vi "VI Tree.vi"   [LabVIEW 2015, in "Agilent 2000 3000 X-Series.lvlib"]
doc: "This is the instrument driver for the Agilent 2000 3000 X-Series oscilloscope. The VI Tree displays all the user-callable VIs of the instrument driver in an organized table."
uses:
  <instrlib>/Agilent 2000 3000 X-Series/Agilent 2000 3000 X-Series.lvlib
  <instrlib>/Agilent 2000 3000 X-Series/Public/Configure/Configure Timebase (Basic).vi
  <instrlib>/Agilent 2000 3000 X-Series/Public/Configure/Configure Measurement Edge (Delay).vi
  <instrlib>/Agilent 2000 3000 X-Series/Public/Action-Status/Reset Count (Mask Test).vi
  <instrlib>/Agilent 2000 3000 X-Series/Public/Configure/Trigger/Configure Trigger (USB).vi
  <instrlib>/Agilent 2000 3000 X-Series/Public/Configure/Serial Bus/Configure Serial Bus (IIC - Trigger).vi
  <instrlib>/Agilent 2000 3000 X-Series/Public/Configure/Reference Waveform/Configure Reference Waveform (Operation).vi
  <instrlib>/Agilent 2000 3000 X-Series/Public/Configure/Math/Configure Math Function (Bus).vi
  <instrlib>/Agilent 2000 3000 X-Series/Public/Configure/Mask Test/Configure Mask Test (Measurement).vi
  <instrlib>/Agilent 2000 3000 X-Series/Public/Configure/Digital Bus/Configure Bus Definition (Bits Mask).vi
  <instrlib>/Agilent 2000 3000 X-Series/Public/Data/Read Waveforms (Single).vi
  <instrlib>/Agilent 2000 3000 X-Series/Public/Data/Read Measurement (Current Value).vi
  <instrlib>/Agilent 2000 3000 X-Series/Public/Data/Read Count Measurement (Event Search).vi
  <instrlib>/Agilent 2000 3000 X-Series/Public/Configure/Event Search/Configure Event Search (Serial Bus - SENT).vi
  <instrlib>/Agilent 2000 3000 X-Series/Public/Configure/Waveform Modulation/Configure Waveform Modulation (AM).vi
  <instrlib>/Agilent 2000 3000 X-Series/Public/Configure/Power Analysis/Configure Power Analysis (Efficiency).vi
  <instrlib>/Agilent 2000 3000 X-Series/Public/Configure/Math/Configure Clock Recovery (Constant Frequency).vi
  <instrlib>/Agilent 2000 3000 X-Series/Public/Data/Read Jitter Measurement (Clock TIE).vi
  <instrlib>/Agilent 2000 3000 X-Series/Public/Configure/Jitter Analysis/Configure Jitter Measurement (N-Period to Period).vi
panel:
  # "(c) 2011-2016 National Instruments.  ALL RIGHTS RESERVED."
  # "SEE DIAGRAM\nFOR VI TREE."
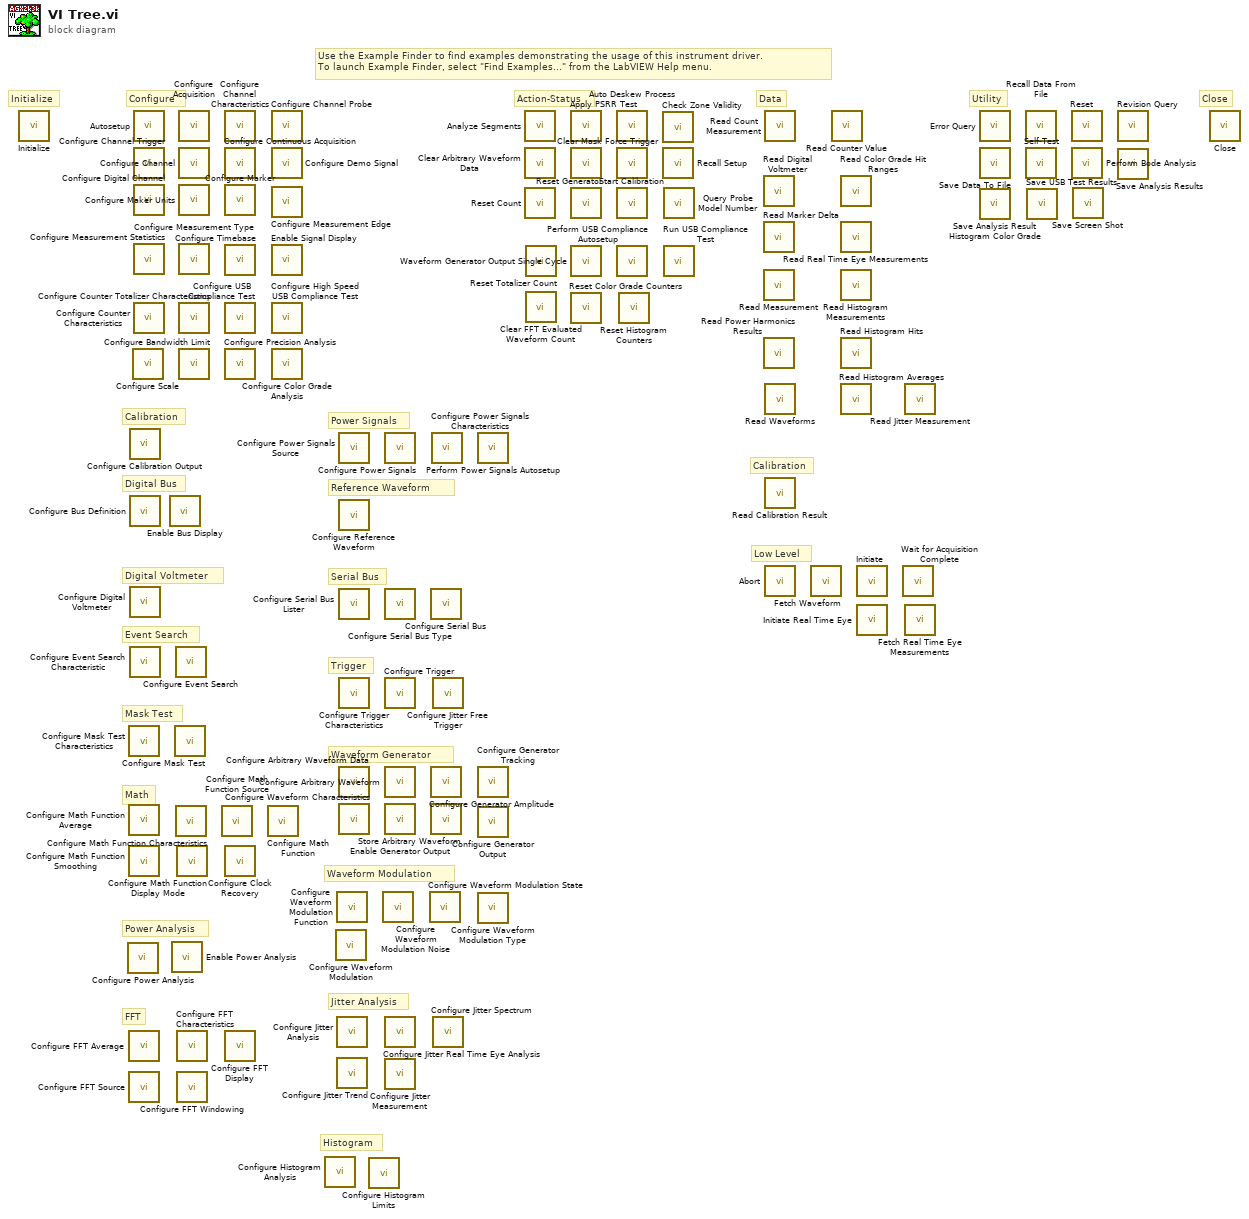
[diagram p0: block diagram]
diagram:
  # "Histogram"
  # "Jitter Analysis"
  # "FFT"
  # "Waveform Modulation"
  # "Digital Voltmeter"
  # "Close"
  # "Utility"
  # "Power Analysis"
  # "Low Level"
  # "Calibration"
  # "Data"
  # "Waveform Generator"
  # "Trigger"
  # "Serial Bus"
  # "Reference Waveform"
  # "Power Signals"
  # "Math"
  # "Mask Test"
  # "Event Search"
  # "Digital Bus"
  # "Calibration"
  # "Configure"
  # "Action-Status"
  # "Initialize"
  # "Use the Example Finder to find examples demonstrating the usage of this instrument driver.\nTo launch Example Finder, select \"Find Examples...\" from the LabVIEW Help menu."
  n1 = call <instrlib>:"Initialize.vi"() -> ()  [unwired: 10 in, 2 out]
  n2 = call-poly <instrlib>:"Configure Power Analysis.vi"() -> ()  [unwired: 10 in, 2 out]
  n3 = call <instrlib>:"Configure Mask Test Characteristics.vi"() -> ()  [unwired: 14 in, 2 out]
  n4 = call <instrlib>:"Configure Math Function Average.vi"() -> ()  [unwired: 10 in, 2 out]
  n5 = call <instrlib>:"Configure Math Function Smoothing.vi"() -> ()  [unwired: 10 in, 2 out]
  n6 = call <instrlib>:"Configure FFT Average.vi"() -> ()  [unwired: 10 in, 2 out]
  n7 = call <instrlib>:"Configure FFT Source.vi"() -> ()  [unwired: 10 in, 2 out]
  n8 = call <instrlib>:"Configure Calibration Output.vi"() -> ()  [unwired: 10 in, 2 out]
  n9 = call-poly <instrlib>:"Configure Bus Definition.vi"() -> ()  [unwired: 10 in, 2 out]
  n10 = call <instrlib>:"Configure Digital Voltmeter.vi"() -> ()  [unwired: 10 in, 2 out]
  n11 = call <instrlib>:"Configure Event Search Characteristic.vi"() -> ()  [unwired: 10 in, 2 out]
  n12 = call <instrlib>:"Configure Scale.vi"() -> ()  [unwired: 10 in, 2 out]
  n13 = call <instrlib>:"Autosetup.vi"() -> ()  [unwired: 10 in, 2 out]
  n14 = call <instrlib>:"Configure Channel Trigger.vi"() -> ()  [unwired: 10 in, 2 out]
  n15 = call <instrlib>:"Configure Digital Channel.vi"() -> ()  [unwired: 10 in, 2 out]
  n16 = call <instrlib>:"Configure Measurement Statistics.vi"() -> ()  [unwired: 10 in, 2 out]
  n17 = call <instrlib>:"Configure Counter Characteristics.vi"() -> ()  [unwired: 14 in, 2 out]
  n18 = call <instrlib>:"Enable Bus Display.vi"() -> ()  [unwired: 10 in, 2 out]
  n19 = call <instrlib>:"Enable Power Analysis.vi"() -> ()  [unwired: 10 in, 2 out]
  n20 = call-poly <instrlib>:"Configure Mask Test.vi"() -> ()  [unwired: 14 in, 2 out]
  n21 = call-poly <instrlib>:"Configure Event Search.vi"() -> ()  [unwired: 10 in, 2 out]
  n22 = call <instrlib>:"Configure Math Function Characteristics.vi"() -> ()  [unwired: 14 in, 2 out]
  n23 = call <instrlib>:"Configure Math Function Display Mode.vi"() -> ()  [unwired: 10 in, 2 out]
  n24 = call <instrlib>:"Configure FFT Characteristics.vi"() -> ()  [unwired: 14 in, 2 out]
  n25 = call <instrlib>:"Configure FFT Windowing.vi"() -> ()  [unwired: 10 in, 2 out]
  n26 = call <instrlib>:"Configure Acquisition.vi"() -> ()  [unwired: 10 in, 2 out]
  n27 = call <instrlib>:"Configure Channel.vi"() -> ()  [unwired: 14 in, 2 out]
  n28 = call <instrlib>:"Configure Maker Units.vi"() -> ()  [unwired: 10 in, 2 out]
  n29 = call <instrlib>:"Configure Measurement Type.vi"() -> ()  [unwired: 14 in, 2 out]
  n30 = call <instrlib>:"Configure Counter Totalizer Characteristics.vi"() -> ()  [unwired: 14 in, 2 out]
  n31 = call <instrlib>:"Configure Bandwidth Limit.vi"() -> ()  [unwired: 10 in, 2 out]
  n32 = call <instrlib>:"Configure Math Function Source.vi"() -> ()  [unwired: 10 in, 2 out]
  n33 = call <instrlib>:"Configure Channel Characteristics.vi"() -> ()  [unwired: 10 in, 2 out]
  n34 = call <instrlib>:"Configure Continuous Acquisition.vi"() -> ()  [unwired: 10 in, 2 out]
  n35 = call <instrlib>:"Configure Marker.vi"() -> ()  [unwired: 14 in, 2 out]
  n36 = call-poly <instrlib>:"Configure Timebase.vi"() -> ()  [unwired: 14 in, 2 out]
  n37 = call <instrlib>:"Configure USB Compliance Test.vi"() -> ()  [unwired: 10 in, 2 out]
  n38 = call <instrlib>:"Configure Precision Analysis.vi"() -> ()  [unwired: 10 in, 2 out]
  n39 = call-poly <instrlib>:"Configure Clock Recovery.vi"() -> ()  [unwired: 10 in, 2 out]
  n40 = call <instrlib>:"Configure FFT Display.vi"() -> ()  [unwired: 10 in, 2 out]
  n41 = call-poly <instrlib>:"Configure Math Function.vi"() -> ()  [unwired: 10 in, 2 out]
  n42 = call <instrlib>:"Configure Channel Probe.vi"() -> ()  [unwired: 10 in, 2 out]
  n43 = call <instrlib>:"Configure Demo Signal.vi"() -> ()  [unwired: 10 in, 2 out]
  n44 = call-poly <instrlib>:"Configure Measurement Edge.vi"() -> ()  [unwired: 10 in, 2 out]
  n45 = call <instrlib>:"Enable Signal Display.vi"() -> ()  [unwired: 10 in, 2 out]
  n46 = call <instrlib>:"Configure High Speed USB Compliance Test.vi"() -> ()  [unwired: 10 in, 2 out]
  n47 = call <instrlib>:"Configure Color Grade Analysis .vi"() -> ()  [unwired: 10 in, 2 out]
  n48 = call <instrlib>:"Configure Histogram Analysis.vi"() -> ()  [unwired: 10 in, 2 out]
  n49 = call-poly <instrlib>:"Configure Waveform Modulation.vi"() -> ()  [unwired: 10 in, 2 out]
  n50 = call <instrlib>:"Configure Waveform Modulation Function.vi"() -> ()  [unwired: 10 in, 2 out]
  n51 = call <instrlib>:"Configure Jitter Analysis.vi"() -> ()  [unwired: 10 in, 2 out]
  n52 = call <instrlib>:"Configure Jitter Trend.vi"() -> ()  [unwired: 10 in, 2 out]
  n53 = call <instrlib>:"Configure Power Signals Source.vi"() -> ()  [unwired: 10 in, 2 out]
  n54 = call-poly <instrlib>:"Configure Reference Waveform.vi"() -> ()  [unwired: 10 in, 2 out]
  n55 = call <instrlib>:"Configure Serial Bus Lister.vi"() -> ()  [unwired: 10 in, 2 out]
  n56 = call <instrlib>:"Configure Trigger Characteristics.vi"() -> ()  [unwired: 14 in, 2 out]
  n57 = call <instrlib>:"Configure Arbitrary Waveform Data.vi"() -> ()  [unwired: 10 in, 2 out]
  n58 = call <instrlib>:"Configure Waveform Characteristics.vi"() -> ()  [unwired: 14 in, 2 out]
  n59 = call <instrlib>:"Configure Histogram Limits.vi"() -> ()  [unwired: 10 in, 2 out]
  n60 = call <instrlib>:"Configure Waveform Modulation Noise.vi"() -> ()  [unwired: 10 in, 2 out]
  n61 = call <instrlib>:"Configure Power Signals.vi"() -> ()  [unwired: 14 in, 2 out]
  n62 = call <instrlib>:"Configure Serial Bus Type.vi"() -> ()  [unwired: 10 in, 2 out]
  n63 = call-poly <instrlib>:"Configure Trigger.vi"() -> ()  [unwired: 10 in, 2 out]
  n64 = call <instrlib>:"Configure Arbitrary Waveform.vi"() -> ()  [unwired: 10 in, 2 out]
  n65 = call <instrlib>:"Enable Generator Output.vi"() -> ()  [unwired: 10 in, 2 out]
  n66 = call <instrlib>:"Configure Jitter Real Time Eye Analysis.vi"() -> ()  [unwired: 10 in, 2 out]
  n67 = call-poly <instrlib>:"Configure Jitter Measurement.vi"() -> ()  [unwired: 10 in, 2 out]
  n68 = call <instrlib>:"Configure Waveform Modulation State.vi"() -> ()  [unwired: 10 in, 2 out]
  n69 = call-poly <instrlib>:"Configure Serial Bus.vi"() -> ()  [unwired: 14 in, 2 out]
  n70 = call <instrlib>:"Configure Generator Amplitude.vi"() -> ()  [unwired: 14 in, 2 out]
  n71 = call <instrlib>:"Store Arbitrary Waveform.vi"() -> ()  [unwired: 10 in, 2 out]
  n72 = call <instrlib>:"Configure Power Signals Characteristics.vi"() -> ()  [unwired: 14 in, 2 out]
  n73 = call <instrlib>:"Configure Jitter Free Trigger.vi"() -> ()  [unwired: 10 in, 2 out]
  n74 = call <instrlib>:"Configure Jitter Spectrum.vi"() -> ()  [unwired: 14 in, 2 out]
  n75 = call <instrlib>:"Perform Power Signals Autosetup.vi"() -> ()  [unwired: 10 in, 2 out]
  n76 = call <instrlib>:"Configure Generator Tracking.vi"() -> ()  [unwired: 10 in, 2 out]
  n77 = call <instrlib>:"Configure Generator Output.vi"() -> ()  [unwired: 10 in, 2 out]
  n78 = call <instrlib>:"Configure Waveform Modulation Type.vi"() -> ()  [unwired: 10 in, 2 out]
  n79 = call <instrlib>:"Analyze Segments.vi"() -> ()  [unwired: 10 in, 2 out]
  n80 = call <instrlib>:"Clear Arbitrary Waveform Data.vi"() -> ()  [unwired: 10 in, 2 out]
  n81 = call-poly <instrlib>:"Reset Count.vi"() -> ()  [unwired: 10 in, 2 out]
  n82 = call <instrlib>:"Reset Totalizer Count.vi"() -> ()  [unwired: 10 in, 2 out]
  n83 = call <instrlib>:"Clear FFT Evaluated Waveform Count.vi"() -> ()  [unwired: 10 in, 2 out]
  n84 = call <instrlib>:"Apply PSRR Test.vi"() -> ()  [unwired: 10 in, 2 out]
  n85 = call <instrlib>:"Clear Mask.vi"() -> ()  [unwired: 10 in, 2 out]
  n86 = call <instrlib>:"Reset Generator.vi"() -> ()  [unwired: 10 in, 2 out]
  n87 = call <instrlib>:"Waveform Generator Output Single Cycle.vi"() -> ()  [unwired: 14 in, 2 out]
  n88 = call <instrlib>:"Reset Color Grade Counters.vi"() -> ()  [unwired: 10 in, 2 out]
  n89 = call <instrlib>:"Auto Deskew Process.vi"() -> ()  [unwired: 10 in, 2 out]
  n90 = call <instrlib>:"Force Trigger.vi"() -> ()  [unwired: 10 in, 2 out]
  n91 = call <instrlib>:"Start Calibration.vi"() -> ()  [unwired: 10 in, 2 out]
  n92 = call <instrlib>:"Perform USB Compliance Autosetup.vi"() -> ()  [unwired: 10 in, 2 out]
  n93 = call <instrlib>:"Reset Histogram Counters.vi"() -> ()  [unwired: 10 in, 2 out]
  n94 = call <instrlib>:"Check Zone Validity.vi"() -> ()  [unwired: 9 in, 3 out]
  n95 = call <instrlib>:"Recall Setup.vi"() -> ()  [unwired: 10 in, 2 out]
  n96 = call <instrlib>:"Query Probe Model Number.vi"() -> ()  [unwired: 13 in, 3 out]
  n97 = call <instrlib>:"Run USB Compliance Test.vi"() -> ()  [unwired: 10 in, 2 out]
  n98 = call <instrlib>:"Read Digital Voltmeter.vi"() -> ()  [unwired: 8 in, 4 out]
  n99 = call <instrlib>:"Read Marker Delta.vi"() -> ()  [unwired: 8 in, 4 out]
  n100 = call-poly <instrlib>:"Read Measurement.vi"() -> ()  [unwired: 13 in, 3 out]
  n101 = call <instrlib>:"Read Power Harmonics Results.vi"() -> ()  [unwired: 9 in, 3 out]
  n102 = call-poly <instrlib>:"Read Count Measurement.vi"() -> ()  [unwired: 9 in, 3 out]
  n103 = call-poly <instrlib>:"Read Waveforms.vi"() -> ()  [unwired: 9 in, 3 out]
  n104 = call <instrlib>:"Read Calibration Result.vi"() -> ()  [unwired: 6 in, 6 out]
  n105 = call <instrlib>:"Abort.vi"() -> ()  [unwired: 10 in, 2 out]
  n106 = call <instrlib>:"Fetch Waveform.vi"() -> ()  [unwired: 9 in, 3 out]
  n107 = call <instrlib>:"Read Counter Value.vi"() -> ()  [unwired: 13 in, 3 out]
  n108 = call <instrlib>:"Read Color Grade Hit Ranges.vi"() -> ()  [unwired: 9 in, 3 out]
  n109 = call <instrlib>:"Read Real Time Eye Measurements.vi"() -> ()  [unwired: 7 in, 5 out]
  n110 = call <instrlib>:"Read Histogram Measurements.vi"() -> ()  [unwired: 9 in, 7 out]
  n111 = call <instrlib>:"Read Histogram Hits.vi"() -> ()  [unwired: 9 in, 7 out]
  n112 = call <instrlib>:"Read Histogram Averages.vi"() -> ()  [unwired: 7 in, 5 out]
  n113 = call <instrlib>:"Initiate.vi"() -> ()  [unwired: 10 in, 2 out]
  n114 = call <instrlib>:"Initiate Real Time Eye.vi"() -> ()  [unwired: 10 in, 2 out]
  n115 = call <instrlib>:"Wait for Acquisition Complete.vi"() -> ()  [unwired: 10 in, 2 out]
  n116 = call-poly <instrlib>:"Read Jitter Measurement.vi"() -> ()  [unwired: 9 in, 3 out]
  n117 = call <instrlib>:"Fetch Real Time Eye Measurements.vi"() -> ()  [unwired: 7 in, 5 out]
  n118 = call <instrlib>:"Error Query.vi"() -> ()  [unwired: 8 in, 4 out]
  n119 = call <instrlib>:"Save Data To File.vi"() -> ()  [unwired: 14 in, 2 out]
  n120 = call <instrlib>:"Save Analysis Result Histogram Color Grade.vi"() -> ()  [unwired: 10 in, 2 out]
  n121 = call <instrlib>:"Recall Data From File.vi"() -> ()  [unwired: 10 in, 2 out]
  n122 = call <instrlib>:"Self-Test.vi"() -> ()  [unwired: 8 in, 4 out]
  n123 = call <instrlib>:"Save USB Test Results.vi"() -> ()  [unwired: 10 in, 2 out]
  n124 = call <instrlib>:"Reset.vi"() -> ()  [unwired: 10 in, 2 out]
  n125 = call <instrlib>:"Perform Bode Analysis.vi"() -> ()  [unwired: 10 in, 2 out]
  n126 = call <instrlib>:"Save Screen Shot.vi"() -> ()  [unwired: 10 in, 2 out]
  n127 = call <instrlib>:"Revision Query.vi"() -> ()  [unwired: 8 in, 4 out]
  n128 = call <instrlib>:"Save Analysis Results.vi"() -> ()  [unwired: 14 in, 2 out]
  n129 = call <instrlib>:"Close.vi"() -> ()  [unwired: 11 in, 1 out]
